vi "GyroscopeStart.vi"(0 "Device Info":T1={"Serial Number"=-1, "Channel"=0, "Port"=0}, 1 "Data Interval":i32=-1, 11 "error in (no error)":errorcluster, 12 "Connection":u16(ring) items=["No Preference", "Remote", "Local"], 13 "Timeout (mSec)":i32=5000) -> (4 "Phidget ID":u64, 6 "Serial Number Return":i32, 10 "Attached?":bool, 15 "error out":errorcluster)   [LabVIEW 2020, in "Phidget Gyroscope.lvlib"]
doc: "${Gyroscope:StartHeader}"
uses:
  <instrlib>/Phidgets/Phidget Gyroscope/Phidget Gyroscope.lvlib
  <instrlib>/Phidgets/Phidget Common/Phidget Common.lvlib
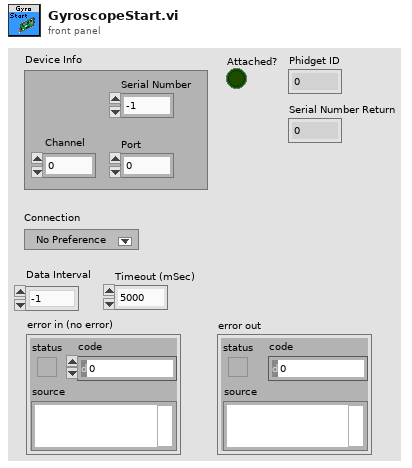
[diagram p1: front panel]
types:
  T1 = cluster{"Serial Number":i32, "Channel":i32, "Port":i32}
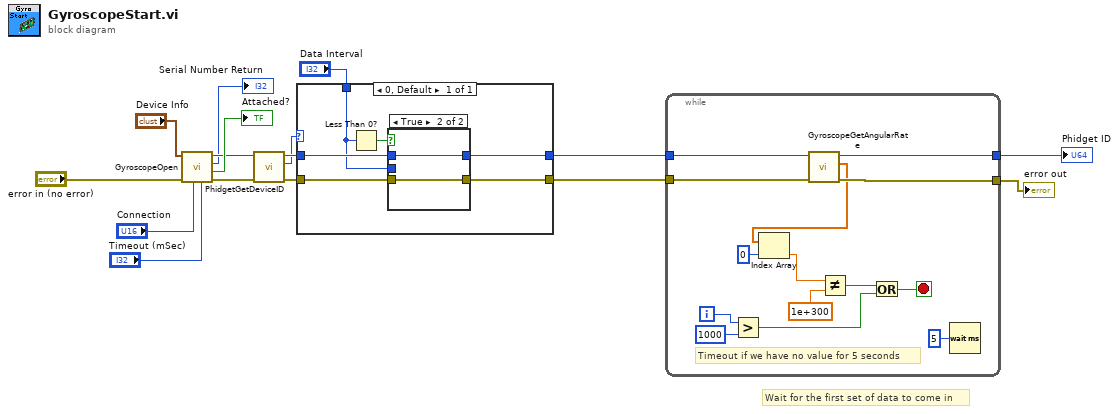
[diagram p0: block diagram]
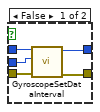
[diagram p2: hidden frame]
diagram:
  # "Wait for the first set of data to come in"
  n1 = call <instrlib>:"GyroscopeOpen.vi"("Timeout (mSec)"="Timeout (mSec)", "Connection"="Connection", "error in"="error in (no error)", "Device Info"="Device Info") -> ("error out"=w13:errorcluster, "Attached?"=→"Attached?":bool, "Serial Number Return"=→"Serial Number Return":i32, "Phidget ID"=w12:u64)  [unwired: 4 in]
  n2 = call <instrlib>:"PhidgetGetDeviceID.vi"("error in (no error)"=w13, "Device In"=w12) -> ("error out"=w10:errorcluster, "Devie IDs"=w9:u32, "Device Out"=w11:u64)  [unwired: 6 in]
  n3 = case shown="0, Default" w9 {
    tunnel: w10 -> [w21]
    tunnel: [w18] -> w3
    tunnel: w11 -> [w20]
    tunnel: [w17] -> w4
    tunnel: "Data Interval" -> [w19]
    frame 0, Default {
      n4 = Less Than 0?(x=w19) -> (x < 0?=w22:bool)
      n5 = case shown="True" w22 {
        tunnel: w20 -> [w27 w29]
        tunnel: w21 -> [w26 w28]
        tunnel: [w24 w29] -> w17
        tunnel: [w25 w28] -> w18
        tunnel: w19 -> [w23 _]
        frame False {
          n6 = call <instrlib>:"GyroscopeSetDataInterval.vi"("error in (no error)"=w26, "Interval"=w23, "Device In"=w27) -> ("error out"=w25:errorcluster, "Device Out"=w24:u64)  [unwired: 6 in]
        }
        frame True {
        }
      }
    }
  }
  n7 = while {
    tunnel: w4 -> [w41]
    tunnel: w3 -> [w40]
    tunnel: [w38] -> w8
    tunnel: [w39] -> w15
    i -> [w36]
    stop <- w33 stop-if-true
    # "Timeout if we have no value for 5 seconds"
    n8 = Greater?(x=w36, y=1000) -> (0:w34:bool)
    n9 = call <instrlib>:"GyroscopeGetAngularRate.vi"("error in (no error)"=w40, "Device In"=w41) -> ("error out"=w39:errorcluster, "AngularRate"=w31:dbl[], "Device Out"=w38:u64)  [unwired: 6 in]
    n10 = Index Array(array=w31, index=0) -> (element=w30:dbl)
    n11 = Not Equal?(x=w30, y=1e+300) -> (x != y?=w35:bool)
    n12 = Or(x=w35, y=w34) -> (x .or. y?=w33:bool)
    n13 = Wait (ms)(milliseconds to wait=u32 5) -> ()  [unwired: 1 out]
  }
  "error out" <- w15
  "Phidget ID" <- w8
